vi "calculator.vi"() -> ()   [LabVIEW 2015]
panel:
  out "output array 3":u32[](array[numeric])
  out "Numeric":i32
  out "spreadsheet string 2":string
  out "output array 2":u32[](array[numeric])
  out "output array":u32[](array[numeric])
  in  "OK Button 14":bool
  in  "OK Button 13":bool
  in  "OK Button 12":bool
  in  "OK Button 11":bool
  out "spreadsheet string":string
  in  "OK Button 10":bool
  in  "OK Button 9":bool
  in  "OK Button 8":bool
  in  "OK Button 7":bool
  in  "OK Button 6":bool
  in  "OK Button 5":bool
  in  "OK Button 4":bool
  in  "OK Button 3":bool
  in  "OK Button 2":bool
  in  "OK Button":bool
  in  "stop":bool
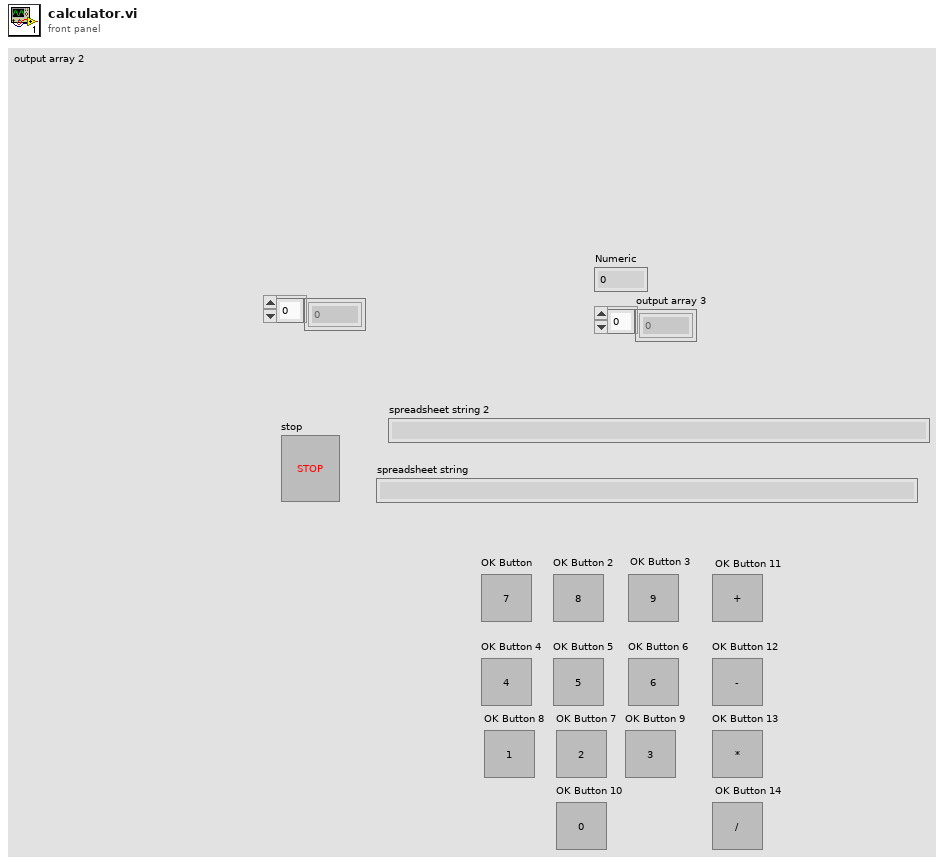
[diagram p1: front panel]
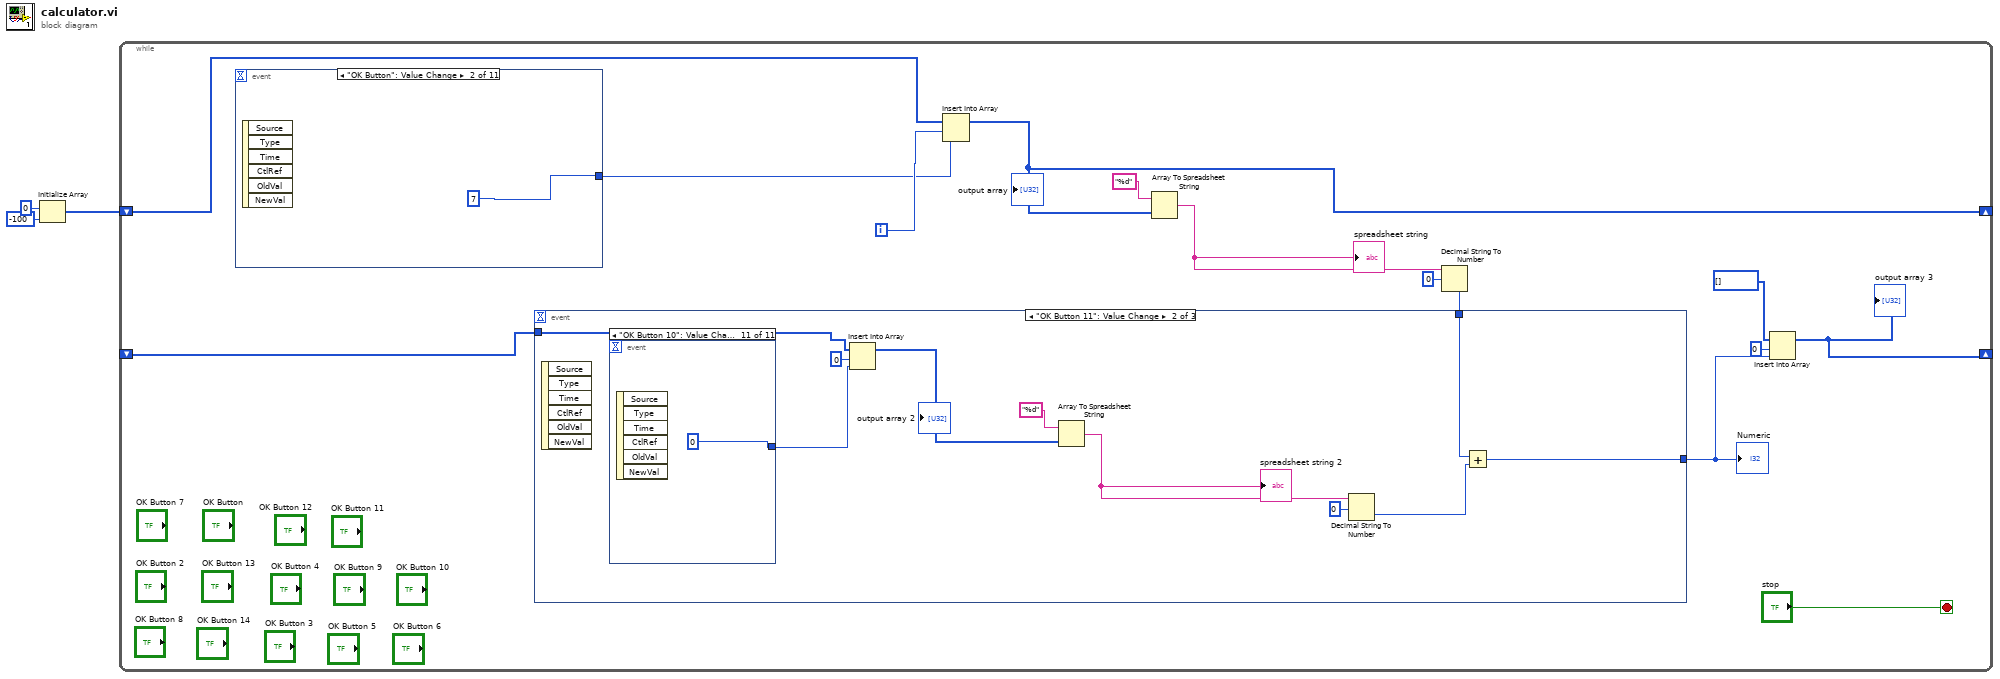
[diagram p0: block diagram]
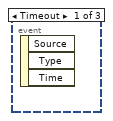
[diagram p2: hidden frame]
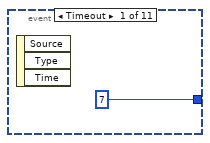
[diagram p3: hidden frame]
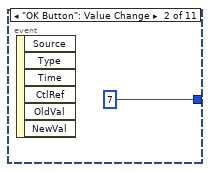
[diagram p4: hidden frame]
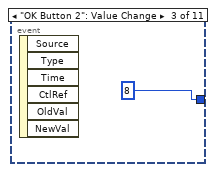
[diagram p5: hidden frame]
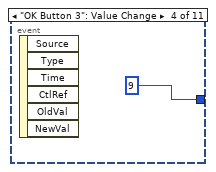
[diagram p6: hidden frame]
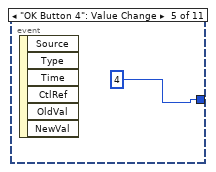
[diagram p7: hidden frame]
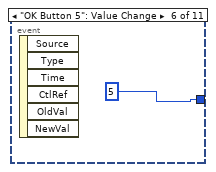
[diagram p8: hidden frame]
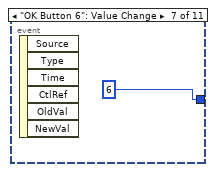
[diagram p9: hidden frame]
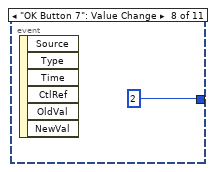
[diagram p10: hidden frame]
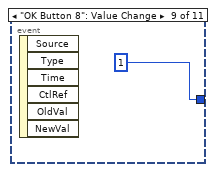
[diagram p11: hidden frame]
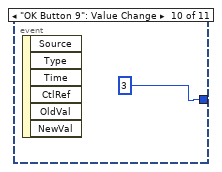
[diagram p12: hidden frame]
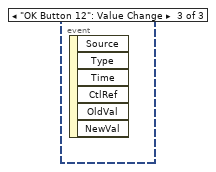
[diagram p13: hidden frame]
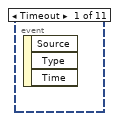
[diagram p14: hidden frame]
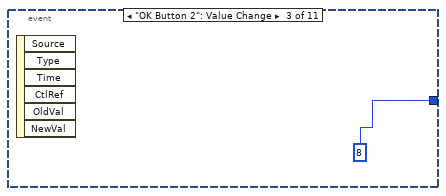
[diagram p15: hidden frame]
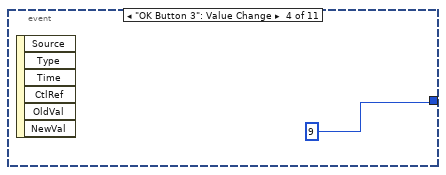
[diagram p16: hidden frame]
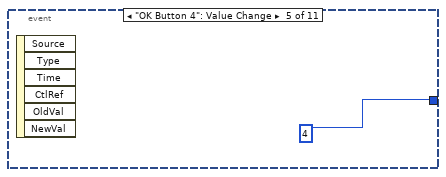
[diagram p17: hidden frame]
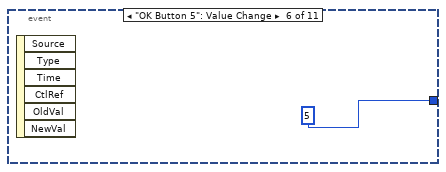
[diagram p18: hidden frame]
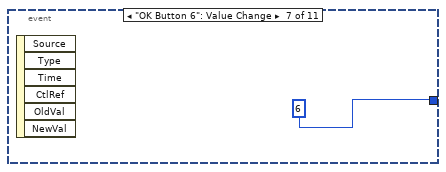
[diagram p19: hidden frame]
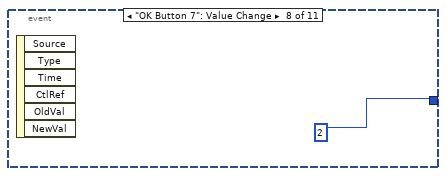
[diagram p20: hidden frame]
diagram:
  n1 = Initialize Array(u32 0 ("element"), -100 ("dimension size")) -> (w1:u32[])
  n2 = while {
    shift-right: [w10] -> _
    shift-left: w1 -> [w9]
    shift-right: [w5] -> _
    shift-left: _ -> [w8]
    i -> [w15]
    stop <- "stop" stop-if-true
    n3 = event shown="[1] \"OK Button\": Value Change" {
      selector: _ -> [_ _ _ _ _ _ _ _ _ _ _]
      dyn-events: _ -> [_ _ _ _ _ _ _ _ _ _ _]
      timeout: _ -> [_ _ _ _ _ _ _ _ _ _ _]
      tunnel: [_ 7 8 9 4 5 6 2 u32 1 3 0] -> w14
      event Timeout {
        n4 = event-data() -> ()  [unwired: 1 in, 3 out]
      }
      event "OK Button": Value Change {
        n5 = event-data() -> ()  [unwired: 1 in, 6 out]
      }
      event "OK Button 2": Value Change {
        n6 = event-data() -> ()  [unwired: 1 in, 6 out]
      }
      event "OK Button 3": Value Change {
        n7 = event-data() -> ()  [unwired: 1 in, 6 out]
      }
      event "OK Button 4": Value Change {
        n8 = event-data() -> ()  [unwired: 1 in, 6 out]
      }
      event "OK Button 5": Value Change {
        n9 = event-data() -> ()  [unwired: 1 in, 6 out]
      }
      event "OK Button 6": Value Change {
        n10 = event-data() -> ()  [unwired: 1 in, 6 out]
      }
      event "OK Button 7": Value Change {
        n11 = event-data() -> ()  [unwired: 1 in, 6 out]
      }
      event "OK Button 8": Value Change {
        n12 = event-data() -> ()  [unwired: 1 in, 6 out]
      }
      event "OK Button 9": Value Change {
        n13 = event-data() -> ()  [unwired: 1 in, 6 out]
      }
      event "OK Button 10": Value Change {
        n14 = event-data() -> ()  [unwired: 1 in, 6 out]
      }
    }
    n15 = Insert Into Array(array=w9, index=w15, new element=w14) -> (w10:u32[])
    "output array" <- w10
    n16 = Array To Spreadsheet String(array=w10, 3:"%d" ("format string")) -> (spreadsheet string=w13:string)  [unwired: 1 in]
    "spreadsheet string" <- w13
    n17 = Decimal String To Number(string=w13, offset=0) -> (number=w12:i32)  [unwired: 1 in, 1 out]
    n18 = event shown="[1] \"OK Button 11\": Value Change" {
      selector: _ -> [_ _ _]
      dyn-events: _ -> [_ _ _]
      timeout: _ -> [_ _ _]
      tunnel: w12 -> [_ w23 _]
      tunnel: [_ w20 _] -> w6
      tunnel: w8 -> [_ w19 _]
      event Timeout {
        n19 = event-data() -> ()  [unwired: 1 in, 3 out]
      }
      event "OK Button 11": Value Change {
        n20 = event-data() -> ()  [unwired: 1 in, 6 out]
        n21 = event shown="[10] \"OK Button 10\": Value Change" {
          selector: _ -> [_ _ _ _ _ _ _ _ _ _ _]
          dyn-events: _ -> [_ _ _ _ _ _ _ _ _ _ _]
          timeout: _ -> [_ _ _ _ _ _ _ _ _ _ _]
          tunnel: [7 7 8 9 4 5 6 2 1 3 0] -> w24
          event Timeout {
            n22 = event-data() -> ()  [unwired: 1 in, 3 out]
          }
          event "OK Button": Value Change {
            n23 = event-data() -> ()  [unwired: 1 in, 6 out]
          }
          event "OK Button 2": Value Change {
            n24 = event-data() -> ()  [unwired: 1 in, 6 out]
          }
          event "OK Button 3": Value Change {
            n25 = event-data() -> ()  [unwired: 1 in, 6 out]
          }
          event "OK Button 4": Value Change {
            n26 = event-data() -> ()  [unwired: 1 in, 6 out]
          }
          event "OK Button 5": Value Change {
            n27 = event-data() -> ()  [unwired: 1 in, 6 out]
          }
          event "OK Button 6": Value Change {
            n28 = event-data() -> ()  [unwired: 1 in, 6 out]
          }
          event "OK Button 7": Value Change {
            n29 = event-data() -> ()  [unwired: 1 in, 6 out]
          }
          event "OK Button 8": Value Change {
            n30 = event-data() -> ()  [unwired: 1 in, 6 out]
          }
          event "OK Button 9": Value Change {
            n31 = event-data() -> ()  [unwired: 1 in, 6 out]
          }
          event "OK Button 10": Value Change {
            n32 = event-data() -> ()  [unwired: 1 in, 6 out]
          }
        }
        n33 = Insert Into Array(array=w19, index=0, new element=w24) -> (w26:u32[])
        "output array 2" <- w26
        n34 = Array To Spreadsheet String(array=w26, 3:"%d" ("format string")) -> (spreadsheet string=w27:string)  [unwired: 1 in]
        "spreadsheet string 2" <- w27
        n35 = Decimal String To Number(string=w27, offset=0) -> (number=w22:i32)  [unwired: 1 in, 1 out]
        n36 = Add(x=w23, y=w22) -> (x+y=w20:i32)
      }
      event "OK Button 12": Value Change {
        n37 = event-data() -> ()  [unwired: 1 in, 6 out]
      }
    }
    "Numeric" <- w6
    n38 = Insert Into Array(array=u32[] [], index=0, new element=w6) -> (w5:u32[])
    "output array 3" <- w5
  }
